vi "PIP_to_JSON.vi"(8 "error in (no error)":errorcluster, 10 "FileName":string) -> (0 "error out":errorcluster)   [LabVIEW 2018]
uses:
  Global Variables.vi
  <vilib>/LVH/i3 JSON/JSON Generation/Create Value Files/Create Value - Object.vi
  <vilib>/LVH/i3 JSON/JSON Generation/Add Object Parameter Files/Add Object Parameter - 1D Array String.vi
  <vilib>/LVH/i3 JSON/i3-json.lvlib
panel:
  out "result string":string
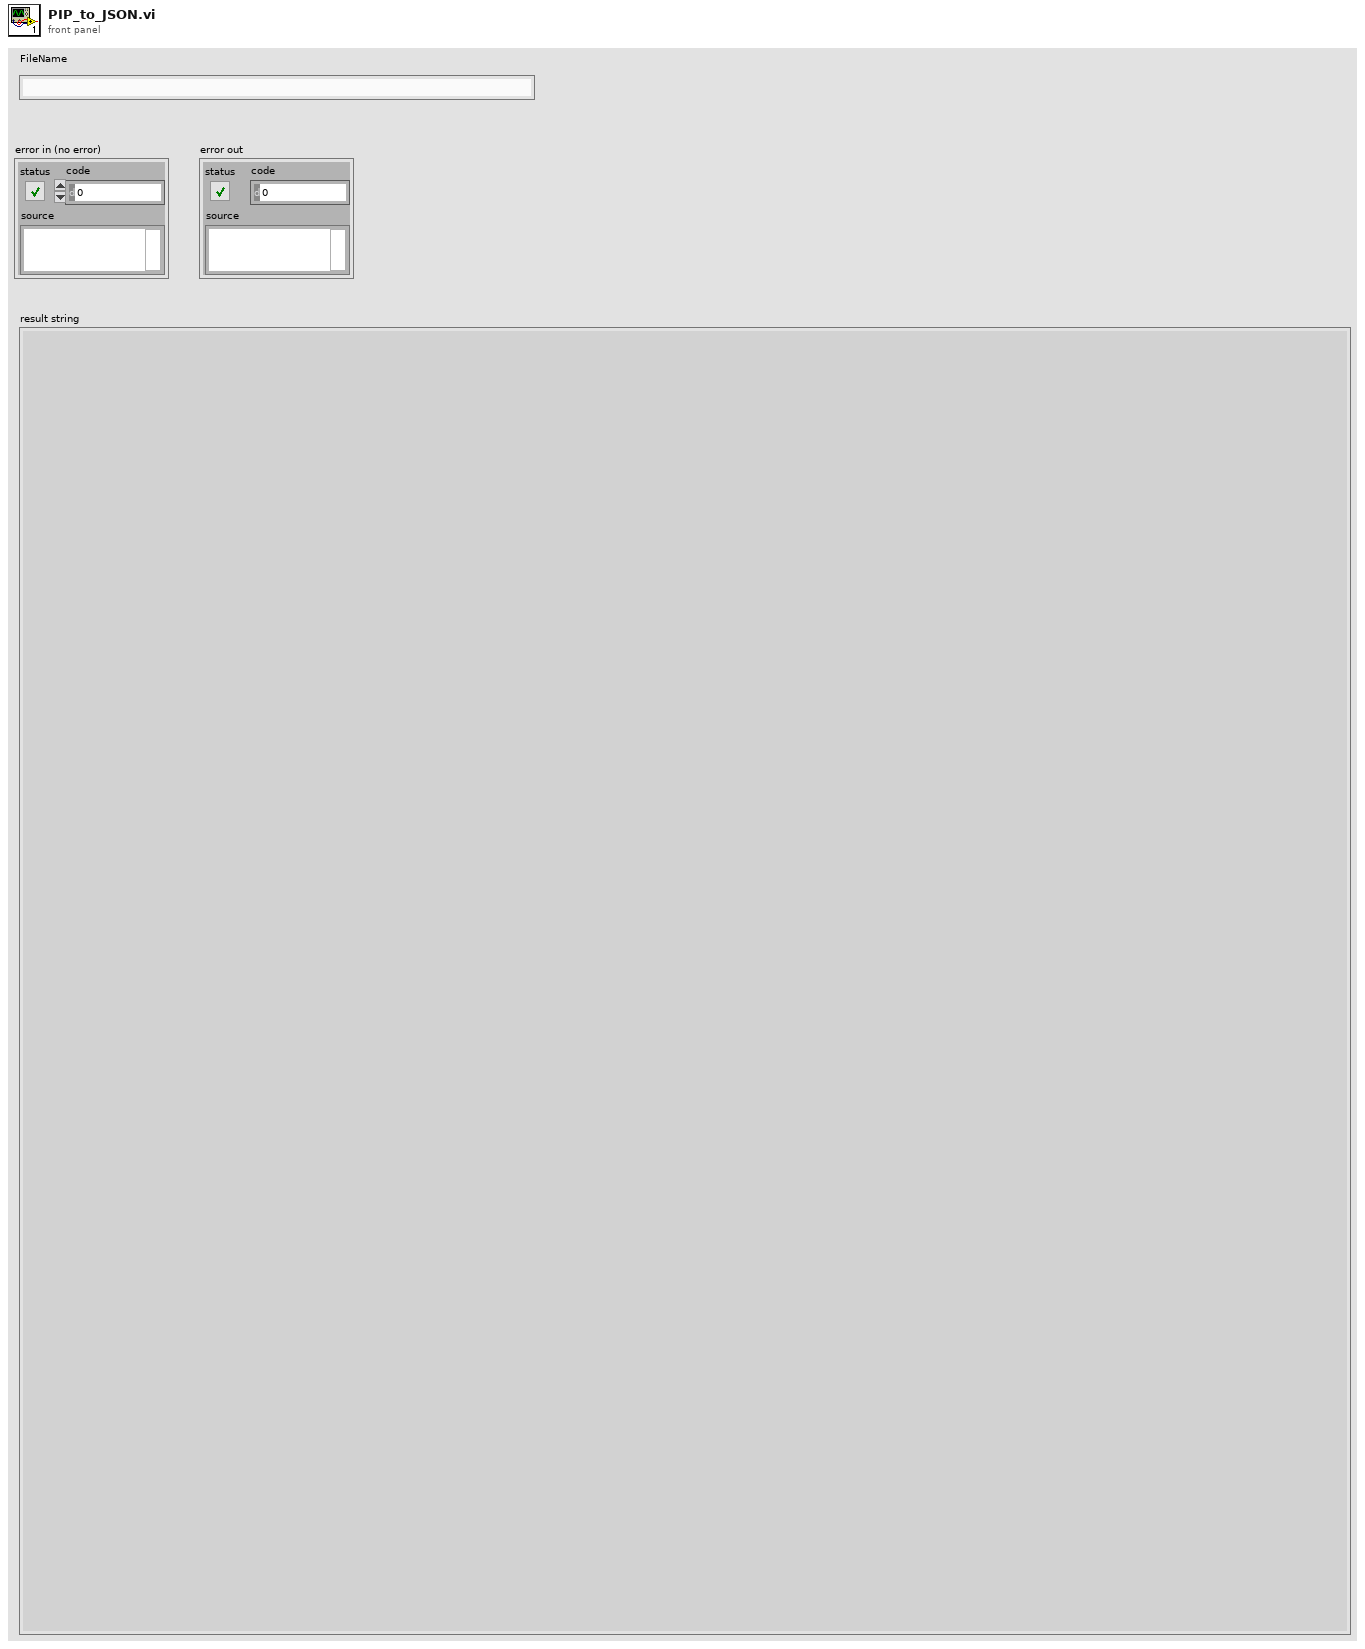
[diagram p1: front panel]
types:
  T1 = enum16{"open", "replace", "create", "open or create", "replace or create", "replace or create with confirmation"}
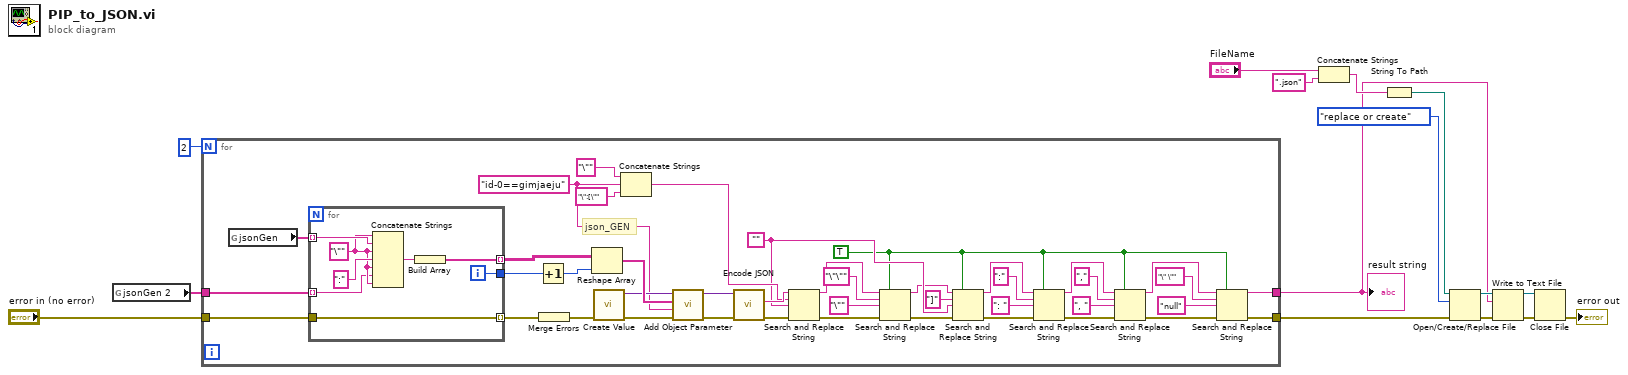
[diagram p0: block diagram]
diagram:
  n1 = global read "Global Variables.vi" "jsonGen 2"() -> (w4:string[])
  n2 = for {
    N: 2 -> [_]
    tunnel: "error in (no error)" -> [w40]
    tunnel: w4 -> [w38]
    tunnel: [w22] -> w3
    tunnel: [w21] -> w2
    w17 = TRUE ("replace all? (F)")
    w46 = ""
    w52 = "id-0==gimjaeju" ("String 2")
    # "json_GEN"
    n3 = global read "Global Variables.vi" "jsonGen"() -> (w56:string[])
    n4 = for {
      tunnel: w56 -> [w65] mode=indexing
      tunnel: [w61] -> w33 mode=indexing
      tunnel: w38 -> [w60] mode=indexing
      tunnel: w40 -> [w59]
      tunnel: [w59] -> w41 mode=indexing
      tunnel: [w58] -> w39
      i -> [w58]
      w63 = "\"" ("string")
      n5 = Concatenate Strings(w63, w65, w63, ":" ("string"), w63, w60, w63) -> (w62:string)
      n6 = Build Array(w62) -> (w61:string[])
    }
    n7 = Increment(x=w39) -> (x+1=w57:i32)
    n8 = Merge Errors(w41) -> (w42:errorcluster)
    n9 = Reshape Array(w33, w57) -> (w54:string[])
    n10 = call-poly <vilib>:"Create Value.vi"("error in (no error)"=w42) -> ("error out"=w43:errorcluster, "JSON Tree"=w53:variant)  [unwired: 9 in]
    n11 = Concatenate Strings("\"" ("string"), w52, "\":[\"" ("string")) -> (w48:string)
    n12 = call-poly <vilib>:"Add Object Parameter.vi"("error in (no error)"=w43, "Name"=w52, "1D String"=w54, "JSON Tree in (JSON Object)"=w53) -> ("error out"=w44:errorcluster, "JSON Tree out (JSON Object)"=w55:variant)  [unwired: 6 in]
    n13 = call <vilib>:"Encode JSON.vi"("error in (no error)"=w44, "JSON Tree"=w55) -> ("error out"=w45:errorcluster, "String"=w49:string)  [unwired: 4 in]
    n14 = Search and Replace String(input string=w49, search string=w48, replace string=w46, error in=w45) -> (result string=w34:string, error out=w37:errorcluster)  [unwired: 4 in, 2 out]
    n15 = Search and Replace String(replace all?=w17, input string=w34, search string="\"\"", replace string="\"", error in=w37) -> (result string=w35:string, error out=w36:errorcluster)  [unwired: 3 in, 2 out]
    n16 = Search and Replace String(replace all?=w17, input string=w35, search string="]", replace string=w46, error in=w36) -> (result string=w25:string, error out=w24:errorcluster)  [unwired: 3 in, 2 out]
    n17 = Search and Replace String(replace all?=w17, input string=w25, search string=":", replace string=": " ("replace string (\"\")"), error in=w24) -> (result string=w30:string, error out=w23:errorcluster)  [unwired: 3 in, 2 out]
    n18 = Search and Replace String(replace all?=w17, input string=w30, search string=",", replace string=", " ("replace string (\"\")"), error in=w23) -> (result string=w18:string, error out=w16:errorcluster)  [unwired: 3 in, 2 out]
    n19 = Search and Replace String(replace all?=w17, input string=w18, search string="\" \"", replace string="null" ("replace string (\"\")"), error in=w16) -> (result string=w22:string, error out=w21:errorcluster)  [unwired: 3 in, 2 out]
  }
  "result string" <- w3
  n20 = Concatenate Strings("FileName", ".json" ("string")) -> (w13:string)
  n21 = String To Path(string=w13) -> (path=w5:path)
  n22 = Open/Create/Replace File(file path (use dialog)=w5, error in=w2, operation (0:open)=T1."replace or create") -> (refnum out=w8:refnum<file>, error out=w7:errorcluster)  [unwired: 3 in, 1 out]
  n23 = Write to Text File(file (use dialog)=w8, text=w3, error in=w7) -> (refnum out=w10:refnum<file>, error out=w9:errorcluster)  [unwired: 1 in, 1 out]
  n24 = Close File(refnum=w10, error in=w9) -> (error out=→"error out":errorcluster)  [unwired: 1 out]
